vi "19.2-FFT.vi"() -> ()   [LabVIEW 2020]
doc: "This example demonstrates how to use the Chirp Z Transform VI to evaluate a partial DFT. Also, it shows how to calculate the starting point and increment for the Chirp Z Transform VI giving the sampling frequency, high frequency, low frequency and number of bins."
uses:
  <vilib>/Analysis/2dsp.llb/Real FFT.vi
  <vilib>/Analysis/NI_AALPro.lvlib
  <vilib>/Analysis/NI_AALBase.lvlib
panel:
  in  "#Samples":dbl=1024.0
  out "F-Im":dbl[](graph) caption="ImX[k]"
  out "F-Re":dbl[](graph) caption="ReX[k]"
  out "F-Phase":dbl[](graph) caption="PhaseX[k]"
  out "F-Amplitude":cluster{dbl, dbl, dbl[]}(graph) caption="MagX[k]"
  out "Signal":waveform(dbl)(graph)
  in  "Stop":bool
  in  "f2 (Hz)":dbl(slide)=20.0 scale=0.0..100.0
  in  "f1 (Hz)":dbl(slide)=200.0 scale=110.0..300.0
  in  "fs (Hz)":dbl=1024.0
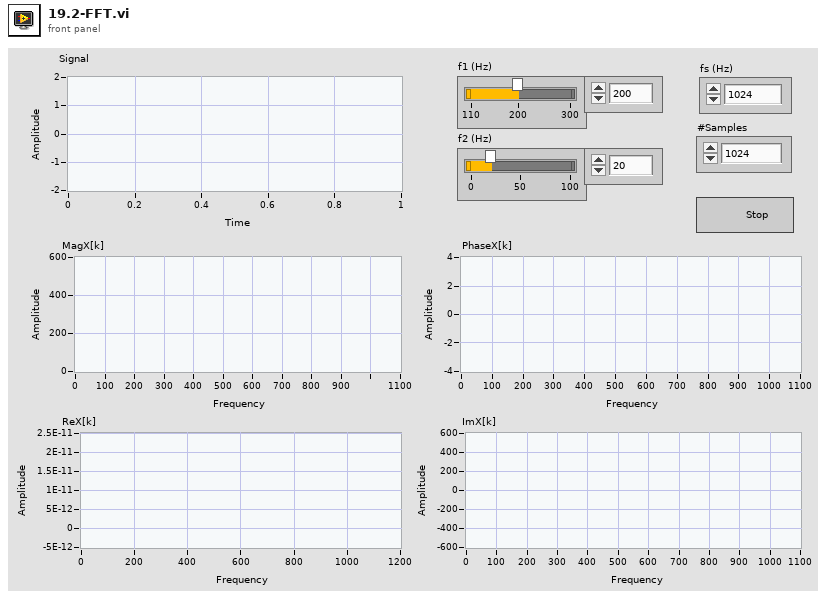
[diagram p1: front panel]
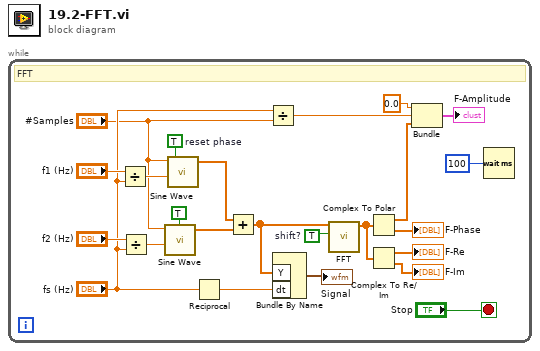
[diagram p0: block diagram]
diagram:
  n1 = while {
    stop <- "Stop" stop-if-true
    w9 = TRUE  # shift?
    w21 = TRUE  # reset phase
    # "FFT"
    n2 = Divide(x="f1 (Hz)", y="fs (Hz)") -> (x/y=w22:dbl)
    n3 = Divide(x="f2 (Hz)", y="fs (Hz)") -> (x/y=w19:dbl)
    n4 = call <vilib>:"Sine Wave.vi"("samples"="#Samples", "frequency"=w19, "reset phase"=TRUE) -> ("sine wave"=w18:dbl[])  [unwired: 2 in, 2 out]
    n5 = call <vilib>:"Sine Wave.vi"("samples"="#Samples", "frequency"=w22, "reset phase"=w21) -> ("sine wave"=w20:dbl[])  [unwired: 2 in, 2 out]
    n6 = Reciprocal(x="fs (Hz)") -> (1/x=w16:dbl)
    n7 = Add(x=w20, y=w18) -> (x+y=w3:dbl[])
    n8 = Divide(x="fs (Hz)", y="#Samples") -> (x/y=w13:dbl)
    n9 = Bundle By Name("Y"=w3, "dt"=w16) -> (→"Signal":waveform(dbl))  [unwired: 1 out]
    n10 = call-poly <vilib>:"FFT.vi"("shift?"=w9, "X"=w3) -> ("FFT {X}"=w6:cdb[])  [unwired: 1 in, 8 out]
    n11 = Complex To Polar(r * e^(i*theta)=w6) -> (r=w8:dbl[], theta=→"F-Phase":dbl[])
    n12 = Complex To Re/Im(x + iy=w6) -> (x=→"F-Re":dbl[], y=→"F-Im":dbl[])
    n13 = Bundle(0.0, w13, w8) -> (→"F-Amplitude":cluster{dbl, dbl, dbl[]})  [unwired: 1 out]
    n14 = Wait (ms)(milliseconds to wait=u32 100) -> ()  [unwired: 1 out]
  }
